vi "1830-C & CM110.vi"() -> (1 "Response":string)   [LabVIEW 2012]
doc: "This VI allows the user to communicate with the 1835-C through the GPIB bus. If the command sent is a query, the VI will automatically read the response. This VI also checks for errors and lets the user know if one exists."
panel:
  out "millisecond timer value":u32
  out "Message String 4":string
  out "1830-C Label on top. 4":string="Optical Power Meter     Model 1830-C"
  out "Power":string
  out "488 Timeout 4":i32
  in  "time delay  2":u32=6000
  out "status byte 2":u8
  out "cancel byte  2":u8 step=1
  out "timeout  2":bool
  in  "NEW GRT?":u8=1 min=1 max=2 step=1
  in  "port number  2":T1(ring)
  in  "1830-C GPIB Address 2":i16=4
  out "1830-C Label on top. 2":string="Optical Power Meter     Model 1830-C"
  out "error out":errorcluster
  in  "error in (no error)":errorcluster
  in  "File":path
  out "Message String 3":string
  out "Wavelength":string
  out "488 Timeout 3":i32
  out "String":string
  in  "WAVELENGTH":u16
  in  "time delay":u32=20000
  out "status byte":u8
  out "cancel byte":u8
  out "timeout":bool
  in  "port number":T1(ring)
  out "488 Timeout":i32
  out "Message String":string
  out "1830-C Label on top.":string="Optical Power Meter     Model 1830-C"
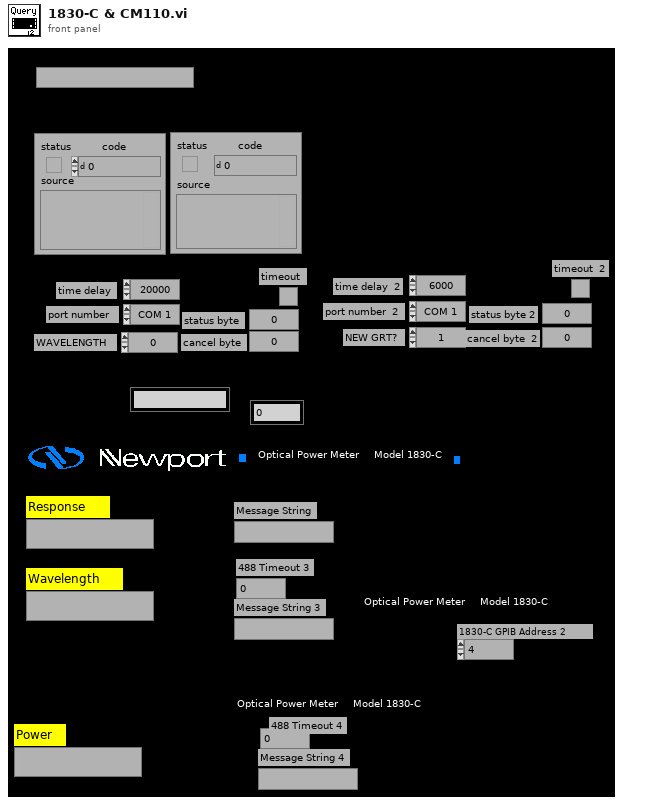
[diagram p1: front panel]
types:
  T1 = enum8{"COM 1", "COM 2", "COM 3", "COM 4", "COM 5", "COM 6", "COM 7", "COM 8", "COM 9"}
  T2 = enum16{"open", "replace", "create", "open or create", "replace or create", "replace or create with confirmation"}
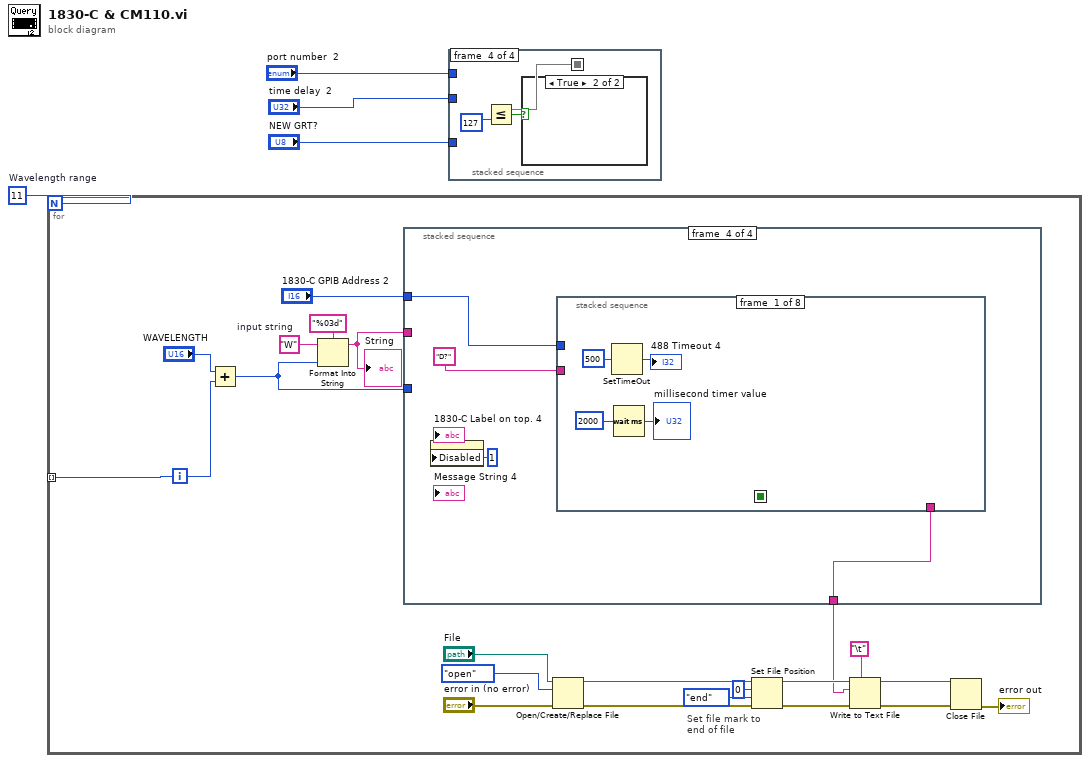
[diagram p0: block diagram]
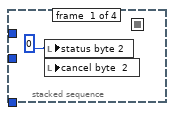
[diagram p2: hidden frame]
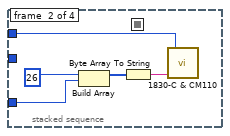
[diagram p3: hidden frame]
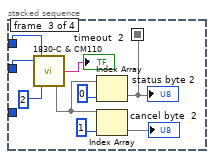
[diagram p4: hidden frame]
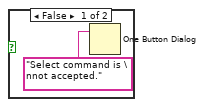
[diagram p5: hidden frame]
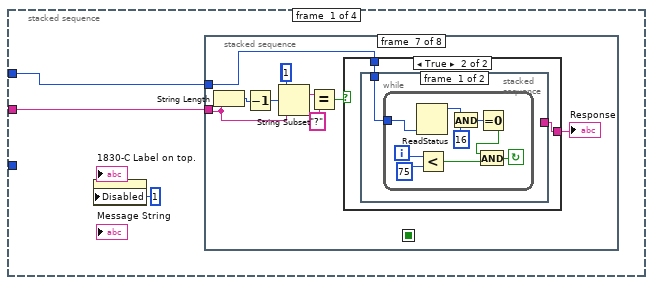
[diagram p6: hidden frame]
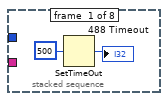
[diagram p7: hidden frame]
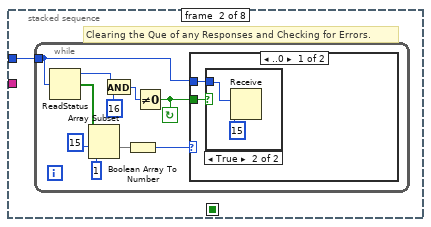
[diagram p8: hidden frame]
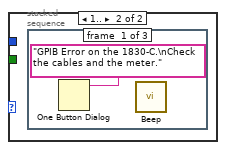
[diagram p10: hidden frame]
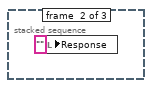
[diagram p11: hidden frame]
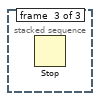
[diagram p12: hidden frame]
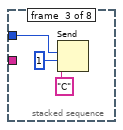
[diagram p13: hidden frame]
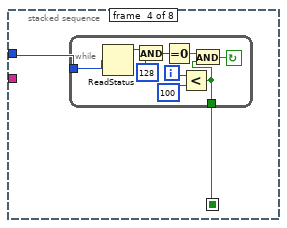
[diagram p14: hidden frame]
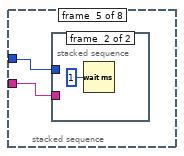
[diagram p15: hidden frame]
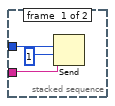
[diagram p16: hidden frame]
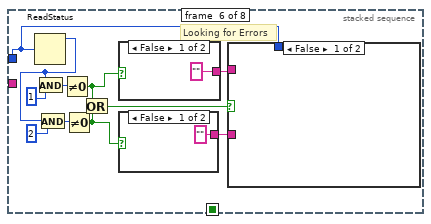
[diagram p17: hidden frame]
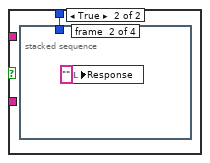
[diagram p18: hidden frame]
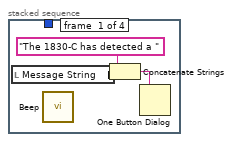
[diagram p19: hidden frame]
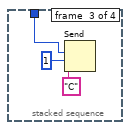
[diagram p20: hidden frame]
diagram:
  w4 = 11  # Wavelength range
  n1 = for {
    N: w4 -> [_]
    tunnel: [w21] -> _ mode=indexing
    i -> [w21]
    w25 = "W"  # input string
    # "Set file mark to\nend of file"
    n2 = Add(x="WAVELENGTH", y=w21) -> (x+y=w20:i32)
    n3 = Format Into String(format string="%03d", initial string=w25, w20) -> (resulting string=w24:string)  [unwired: 1 in, 1 out]
    "String" <- w24
    n4 = stacked-sequence {
      tunnel: w20 -> [_ w117 _ _]
      tunnel: w24 -> [w27 _ _ _]
      tunnel: [_ _ _ w233] -> w6
      tunnel: "1830-C GPIB Address 2" -> [w26 _ w141 w232]
      frame #0 {
        n5 = property on="1830-C Label on top." class="Str"("Disabled"=u8 1) -> ()  [unwired: 2 in, 2 out]
        n6 = stacked-sequence {
          seq-local: [_ _ _ w51 _ _ _ _] -> [_ _ _ _ _ _ _ _]
          tunnel: w27 -> [_ _ _ _ w62 _ w95 _]
          tunnel: w26 -> [_ w31 w49 w52 w63 w68 w99 _]
          frame #0 {
            n7 = SetTimeOut(1:500) -> (0:→"488 Timeout":i32)
          }
          frame #1 {
            # "Clearing the Que of any Responses and Checking for Errors."
            n8 = while {
              tunnel: w31 -> [w33]
              stop <- w35 continue-if-true
              n9 = ReadStatus(4:w33) -> (1:w40:bool[], 2:w34:i16)  [unwired: 2 in, 1 out]
              n10 = Array Subset(array=w40, index=15, length=1) -> (w37:bool[])
              n11 = And(x=w34, y=i16 16) -> (x .and. y?=w41:i16)
              n12 = Boolean Array To Number(Boolean array=w37) -> (number=w36:u32)
              n13 = Not Equal To 0?(x=w41) -> (x != 0?=w35:bool)
              n14 = case shown="..0" w36 {
                tunnel: w35 -> [w43 _]
                tunnel: w33 -> [w42 _]
                frame ..0 {
                  n15 = case shown="True" w43 {
                    tunnel: w42 -> [_ w45]
                    frame False {
                    }
                    frame True {
                      n16 = Receive(6:15, 8:w45) -> ()  [unwired: 3 in, 4 out]
                    }
                  }
                }
                frame 1.. {
                  n17 = stacked-sequence {
                    frame #0 {
                      n18 = One Button Dialog(message="GPIB Error on the 1830-C.\nCheck the cables and the meter.") -> ()  [unwired: 1 in, 1 out]
                      n19 = call <vilib>:"Beep.vi"() -> ()  [unwired: 12 in]
                    }
                    frame #1 {
                      n20 = local write "Response"("") -> ()
                    }
                    frame #2 {
                      n21 = Stop() -> ()  [unwired: 1 in]
                    }
                  }
                }
              }
            }
          }
          frame #2 {
            n22 = Send(2:w49, 3:u8 1, 5:"C") -> ()  [unwired: 2 in, 3 out]
          }
          frame #3 {
            n23 = while {
              tunnel: [w54] -> w51
              tunnel: w52 -> [w53]
              i -> [w57]
              stop <- w55 continue-if-true
              n24 = ReadStatus(4:w53) -> (2:w56:i16)  [unwired: 2 in, 2 out]
              n25 = And(x=w56, y=i16 128) -> (x .and. y?=w60:i16)
              n26 = Equal To 0?(x=w60) -> (x = 0?=w58:bool)
              n27 = Less?(x=w57, y=100) -> (x < y?=w54:bool)
              n28 = And(x=w58, y=w54) -> (x .and. y?=w55:bool)
            }
          }
          frame #4 {
            n29 = stacked-sequence {
              tunnel: w63 -> [w65 _]
              tunnel: w62 -> [w64 _]
              frame #0 {
                n30 = Send(2:w65, 3:u8 1, 5:w64) -> ()  [unwired: 2 in, 3 out]
              }
              frame #1 {
                n31 = Wait (ms)(milliseconds to wait=u32 1) -> ()  [unwired: 1 out]
              }
            }
          }
          frame #5 {
            # "Looking for Errors"
            n32 = ReadStatus(4:w68) -> (2:w76:i16)  [unwired: 2 in, 2 out]
            n33 = And(x=w76, y=i16 1) -> (x .and. y?=w75:i16)
            n34 = And(x=w76, y=i16 2) -> (x .and. y?=w74:i16)
            n35 = Not Equal To 0?(x=w75) -> (x != 0?=w73:bool)
            n36 = Not Equal To 0?(x=w74) -> (x != 0?=w72:bool)
            n37 = Or(x=w73, y=w72) -> (x .or. y?=w71:bool)
            n38 = case shown="False" w73 {
              tunnel: ["" w90] -> w69
              frame False {
              }
              frame True {
                w90 = "Parameter Error."
                n39 = local write "Message String"(w90) -> ()
              }
            }
            n40 = case shown="False" w72 {
              tunnel: ["" w88] -> w70
              frame False {
              }
              frame True {
                w88 = "Command Error."
                n41 = local write "Message String"(w88) -> ()
              }
            }
            n42 = case shown="False" w71 {
              tunnel: w70 -> [_ _]
              tunnel: w69 -> [_ _]
              tunnel: w68 -> [_ w79]
              frame False {
              }
              frame True {
                n43 = stacked-sequence {
                  tunnel: w79 -> [_ _ w84 _]
                  frame #0 {
                    n44 = local read "Message String"() -> (w80:string)
                    n45 = call <vilib>:"Beep.vi"() -> ()  [unwired: 12 in]
                    n46 = Concatenate Strings("The 1830-C has detected a ", w80) -> (w82:string)
                    n47 = One Button Dialog(message=w82) -> ()  [unwired: 1 in, 1 out]
                  }
                  frame #1 {
                    n48 = local write "Response"("") -> ()
                  }
                  frame #2 {
                    n49 = Send(2:w84, 3:u8 1, 5:"C") -> ()  [unwired: 2 in, 3 out]
                  }
                  frame #3 {
                    n50 = Stop() -> ()  [unwired: 1 in]
                  }
                }
              }
            }
          }
          frame #6 {
            (unwired) 1
            n51 = String Length(string=w95) -> (length=w97:i32)
            n52 = Decrement(x=w97) -> (x-1=w96:i32)
            n53 = String Subset(string=w95, offset (0)=w96, length (rest)=1) -> (substring=w94:string)
            n54 = Equal?(x=w94, y="?") -> (x = y?=w92:bool)
            n55 = case shown="True" w92 {
              tunnel: w99 -> [_ w102]
              tunnel: ["" w101] -> w98
              frame False {
              }
              frame True {
                n56 = stacked-sequence {
                  tunnel: w102 -> [w103 w114]
                  tunnel: [_ w113] -> w101
                  frame #0 {
                    n57 = while {
                      tunnel: w103 -> [w109]
                      i -> [w108]
                      stop <- w104 continue-if-true
                      n58 = ReadStatus(4:w109) -> (2:w110:i16)  [unwired: 2 in, 2 out]
                      n59 = Less?(x=w108, y=75) -> (x < y?=w105:bool)
                      n60 = And(x=w110, y=i16 16) -> (x .and. y?=w111:i16)
                      n61 = Equal To 0?(x=w111) -> (x = 0?=w106:bool)
                      n62 = And(x=w106, y=w105) -> (x .and. y?=w104:bool)
                    }
                  }
                  frame #1 {
                    n63 = Receive(6:15, 8:w114) -> (3:w113:string)  [unwired: 3 in, 3 out]
                  }
                }
              }
            }
            "Response" <- w98
          }
          frame #7 {
            n64 = local read "488 Timeout"() -> (w116:i32)
            n65 = SetTimeOut(1:w116) -> ()  [unwired: 1 out]
          }
        }
      }
      frame #1 {
        n66 = stacked-sequence {
          seq-local: [_ _ w131 _] -> [_ _ _ w139]
          tunnel: w117 -> [_ w127 _ _]
          tunnel: "port number" -> [_ w121 w128 _]
          tunnel: "time delay" -> [_ _ w130 _]
          frame #0 {
            w120 = u8 0
            n67 = local write "status byte"(w120) -> ()
            n68 = local write "cancel byte"(w120) -> ()
          }
          frame #1 {
            n69 = Split Number(x=w127) -> (hi(x)=w126:u16, lo(x)=w125:u16)
            n70 = Build Array(u8 16, w126, w125) -> (w123:u16[])
            n71 = Byte Array To String(unsigned byte array=w123) -> (string=w122:string)
            n72 = call "1830-C & CM110.vi"("string to write"=w122, "port number"=w121) -> ()  [unwired: 1 out]
          }
          frame #2 {
            n73 = call "1830-C & CM110.vi"(3:2, 4:w130, 5:w128) -> (0:w133, "Response"=→"timeout":string)  [unwired: 1 in]
            n74 = Index Array(array=w133, index=0) -> (element=w131)
            "status byte" <- w131
            n75 = Index Array(array=w133, index=1) -> (element=→"cancel byte")
          }
          frame #3 {
            n76 = Less Or Equal?(x=w139, y=127) -> (x <= y?=w137:bool)
            n77 = case shown="True" w137 {
              frame False {
                n78 = One Button Dialog(message="Goto command is \nnot accepted.") -> ()  [unwired: 1 in, 1 out]
              }
              frame True {
              }
            }
          }
        }
      }
      frame #2 {
        n79 = property on="1830-C Label on top. 2" class="Str"("Disabled"=u8 1) -> ()  [unwired: 2 in, 2 out]
        n80 = stacked-sequence {
          seq-local: [_ _ _ w166 _ _ _ _] -> [_ _ _ _ _ _ _ _]
          tunnel: "W?" ("Single Command/Query 3") -> [_ _ _ _ w177 _ w211 _]
          tunnel: w141 -> [_ w146 w164 w167 w178 w183 w214 _]
          frame #0 {
            n81 = SetTimeOut(1:500) -> (0:→"488 Timeout 3":i32)
          }
          frame #1 {
            # "Clearing the Que of any Responses and Checking for Errors."
            n82 = while {
              tunnel: w146 -> [w148]
              stop <- w150 continue-if-true
              n83 = ReadStatus(4:w148) -> (1:w155:bool[], 2:w149:i16)  [unwired: 2 in, 1 out]
              n84 = Array Subset(array=w155, index=15, length=1) -> (w152:bool[])
              n85 = And(x=w149, y=i16 16) -> (x .and. y?=w156:i16)
              n86 = Boolean Array To Number(Boolean array=w152) -> (number=w151:u32)
              n87 = Not Equal To 0?(x=w156) -> (x != 0?=w150:bool)
              n88 = case shown="..0" w151 {
                tunnel: w150 -> [w158 _]
                tunnel: w148 -> [w157 _]
                frame ..0 {
                  n89 = case shown="False" w158 {
                    tunnel: w157 -> [_ w160]
                    frame False {
                    }
                    frame True {
                      n90 = Receive(6:15, 8:w160) -> ()  [unwired: 3 in, 4 out]
                    }
                  }
                }
                frame 1.. {
                  n91 = stacked-sequence {
                    frame #0 {
                      n92 = One Button Dialog(message="GPIB Error on the 1830-C.\nCheck the cables and the meter.") -> ()  [unwired: 1 in, 1 out]
                      n93 = call <vilib>:"Beep.vi"() -> ()  [unwired: 12 in]
                    }
                    frame #1 {
                      n94 = local write "Wavelength"("") -> ()
                    }
                    frame #2 {
                      n95 = Stop() -> ()  [unwired: 1 in]
                    }
                  }
                }
              }
            }
          }
          frame #2 {
            n96 = Send(2:w164, 3:u8 1, 5:"C") -> ()  [unwired: 2 in, 3 out]
          }
          frame #3 {
            n97 = while {
              tunnel: [w169] -> w166
              tunnel: w167 -> [w168]
              i -> [w172]
              stop <- w170 continue-if-true
              n98 = ReadStatus(4:w168) -> (2:w171:i16)  [unwired: 2 in, 2 out]
              n99 = And(x=w171, y=i16 128) -> (x .and. y?=w175:i16)
              n100 = Equal To 0?(x=w175) -> (x = 0?=w173:bool)
              n101 = Less?(x=w172, y=100) -> (x < y?=w169:bool)
              n102 = And(x=w173, y=w169) -> (x .and. y?=w170:bool)
            }
          }
          frame #4 {
            n103 = stacked-sequence {
              tunnel: w178 -> [w180 _]
              tunnel: w177 -> [w179 _]
              frame #0 {
                n104 = Send(2:w180, 3:u8 1, 5:w179) -> ()  [unwired: 2 in, 3 out]
              }
              frame #1 {
                n105 = Wait (ms)(milliseconds to wait=u32 1) -> ()  [unwired: 1 out]
              }
            }
          }
          frame #5 {
            # "Looking for Errors"
            n106 = ReadStatus(4:w183) -> (2:w191:i16)  [unwired: 2 in, 2 out]
            n107 = And(x=w191, y=i16 1) -> (x .and. y?=w190:i16)
            n108 = And(x=w191, y=i16 2) -> (x .and. y?=w189:i16)
            n109 = Not Equal To 0?(x=w190) -> (x != 0?=w188:bool)
            n110 = Not Equal To 0?(x=w189) -> (x != 0?=w187:bool)
            n111 = Or(x=w188, y=w187) -> (x .or. y?=w186:bool)
            n112 = case shown="False" w188 {
              tunnel: ["" w205] -> w184
              frame False {
              }
              frame True {
                w205 = "Parameter Error."
                n113 = local write "Message String 3"(w205) -> ()
              }
            }
            n114 = case shown="False" w187 {
              tunnel: ["" w203] -> w185
              frame False {
              }
              frame True {
                w203 = "Command Error."
                n115 = local write "Message String 3"(w203) -> ()
              }
            }
            n116 = case shown="False" w186 {
              tunnel: w185 -> [_ _]
              tunnel: w184 -> [_ _]
              tunnel: w183 -> [_ w194]
              frame False {
              }
              frame True {
                n117 = stacked-sequence {
                  tunnel: w194 -> [_ _ w199 _]
                  frame #0 {
                    n118 = local read "Message String 3"() -> (w195:string)
                    n119 = call <vilib>:"Beep.vi"() -> ()  [unwired: 12 in]
                    n120 = Concatenate Strings("The 1830-C has detected a ", w195) -> (w197:string)
                    n121 = One Button Dialog(message=w197) -> ()  [unwired: 1 in, 1 out]
                  }
                  frame #1 {
                    n122 = local write "Wavelength"("") -> ()
                  }
                  frame #2 {
                    n123 = Send(2:w199, 3:u8 1, 5:"C") -> ()  [unwired: 2 in, 3 out]
                  }
                  frame #3 {
                    n124 = Stop() -> ()  [unwired: 1 in]
                  }
                }
              }
            }
          }
          frame #6 {
            (unwired) 1
            n125 = String Length(string=w211) -> (length=w213:i32)
            n126 = Decrement(x=w213) -> (x-1=w212:i32)
            n127 = String Subset(string=w211, offset (0)=w212, length (rest)=1) -> (substring=w210:string)
            n128 = Equal?(x=w210, y="?") -> (x = y?=w208:bool)
            n129 = case shown="True" w208 {
              tunnel: w214 -> [_ w217]
              tunnel: ["" w216] -> w206
              frame False {
              }
              frame True {
                n130 = stacked-sequence {
                  tunnel: w217 -> [w218 w229]
                  tunnel: [_ w228] -> w216
                  frame #0 {
                    n131 = while {
                      tunnel: w218 -> [w224]
                      i -> [w223]
                      stop <- w219 continue-if-true
                      n132 = ReadStatus(4:w224) -> (2:w225:i16)  [unwired: 2 in, 2 out]
                      n133 = Less?(x=w223, y=75) -> (x < y?=w220:bool)
                      n134 = And(x=w225, y=i16 16) -> (x .and. y?=w226:i16)
                      n135 = Equal To 0?(x=w226) -> (x = 0?=w221:bool)
                      n136 = And(x=w221, y=w220) -> (x .and. y?=w219:bool)
                    }
                  }
                  frame #1 {
                    n137 = Receive(6:15, 8:w229) -> (3:w228:string)  [unwired: 3 in, 3 out]
                  }
                }
              }
            }
            "Wavelength" <- w206
          }
          frame #7 {
            n138 = local read "488 Timeout 3"() -> (w231:i32)
            n139 = SetTimeOut(1:w231) -> ()  [unwired: 1 out]
          }
        }
      }
      frame #3 {
        n140 = property on="1830-C Label on top. 4" class="Str"("Disabled"=u8 1) -> ()  [unwired: 2 in, 2 out]
        n141 = stacked-sequence {
          seq-local: [_ _ _ w260 _ _ _ _] -> [_ _ _ _ _ _ _ _]
          tunnel: "D?" ("Single Command/Query 2") -> [_ _ _ _ w271 _ w305 _]
          tunnel: w232 -> [_ w240 w258 w261 w272 w277 w308 _]
          tunnel: [_ _ _ _ _ _ w300 _] -> w233
          frame #0 {
            n142 = SetTimeOut(1:500) -> (0:→"488 Timeout 4":i32)
            n143 = Wait (ms)(milliseconds to wait=2000) -> (millisecond timer value=→"millisecond timer value":u32)
          }
          frame #1 {
            # "Clearing the Que of any Responses and Checking for Errors."
            n144 = while {
              tunnel: w240 -> [w242]
              stop <- w244 continue-if-true
              n145 = ReadStatus(4:w242) -> (1:w249:bool[], 2:w243:i16)  [unwired: 2 in, 1 out]
              n146 = Array Subset(array=w249, index=15, length=1) -> (w246:bool[])
              n147 = And(x=w243, y=i16 16) -> (x .and. y?=w250:i16)
              n148 = Boolean Array To Number(Boolean array=w246) -> (number=w245:u32)
              n149 = Not Equal To 0?(x=w250) -> (x != 0?=w244:bool)
              n150 = case shown="..0" w245 {
                tunnel: w244 -> [w252 _]
                tunnel: w242 -> [w251 _]
                frame ..0 {
                  n151 = case shown="False" w252 {
                    tunnel: w251 -> [_ w254]
                    frame False {
                    }
                    frame True {
                      n152 = Receive(6:15, 8:w254) -> ()  [unwired: 3 in, 4 out]
                    }
                  }
                }
                frame 1.. {
                  n153 = stacked-sequence {
                    frame #0 {
                      n154 = One Button Dialog(message="GPIB Error on the 1830-C.\nCheck the cables and the meter.") -> ()  [unwired: 1 in, 1 out]
                      n155 = call <vilib>:"Beep.vi"() -> ()  [unwired: 12 in]
                    }
                    frame #1 {
                      n156 = local write "Power"("") -> ()
                    }
                    frame #2 {
                      n157 = Stop() -> ()  [unwired: 1 in]
                    }
                  }
                }
              }
            }
          }
          frame #2 {
            n158 = Send(2:w258, 3:u8 1, 5:"C") -> ()  [unwired: 2 in, 3 out]
          }
          frame #3 {
            n159 = while {
              tunnel: [w263] -> w260
              tunnel: w261 -> [w262]
              i -> [w266]
              stop <- w264 continue-if-true
              n160 = ReadStatus(4:w262) -> (2:w265:i16)  [unwired: 2 in, 2 out]
              n161 = And(x=w265, y=i16 128) -> (x .and. y?=w269:i16)
              n162 = Equal To 0?(x=w269) -> (x = 0?=w267:bool)
              n163 = Less?(x=w266, y=100) -> (x < y?=w263:bool)
              n164 = And(x=w267, y=w263) -> (x .and. y?=w264:bool)
            }
          }
          frame #4 {
            n165 = stacked-sequence {
              tunnel: w272 -> [w274 _]
              tunnel: w271 -> [w273 _]
              frame #0 {
                n166 = Send(2:w274, 3:u8 1, 5:w273) -> ()  [unwired: 2 in, 3 out]
              }
              frame #1 {
                n167 = Wait (ms)(milliseconds to wait=u32 1) -> ()  [unwired: 1 out]
              }
            }
          }
          frame #5 {
            # "Looking for Errors"
            n168 = ReadStatus(4:w277) -> (2:w285:i16)  [unwired: 2 in, 2 out]
            n169 = And(x=w285, y=i16 1) -> (x .and. y?=w284:i16)
            n170 = And(x=w285, y=i16 2) -> (x .and. y?=w283:i16)
            n171 = Not Equal To 0?(x=w284) -> (x != 0?=w282:bool)
            n172 = Not Equal To 0?(x=w283) -> (x != 0?=w281:bool)
            n173 = Or(x=w282, y=w281) -> (x .or. y?=w280:bool)
            n174 = case shown="False" w282 {
              tunnel: ["" w299] -> w278
              frame False {
              }
              frame True {
                w299 = "Parameter Error."
                n175 = local write "Message String 4"(w299) -> ()
              }
            }
            n176 = case shown="False" w281 {
              tunnel: ["" w297] -> w279
              frame False {
              }
              frame True {
                w297 = "Command Error."
                n177 = local write "Message String 4"(w297) -> ()
              }
            }
            n178 = case shown="False" w280 {
              tunnel: w279 -> [_ _]
              tunnel: w278 -> [_ _]
              tunnel: w277 -> [_ w288]
              frame False {
              }
              frame True {
                n179 = stacked-sequence {
                  tunnel: w288 -> [_ _ w293 _]
                  frame #0 {
                    n180 = local read "Message String 4"() -> (w289:string)
                    n181 = call <vilib>:"Beep.vi"() -> ()  [unwired: 12 in]
                    n182 = Concatenate Strings("The 1830-C has detected a ", w289) -> (w291:string)
                    n183 = One Button Dialog(message=w291) -> ()  [unwired: 1 in, 1 out]
                  }
                  frame #1 {
                    n184 = local write "Power"("") -> ()
                  }
                  frame #2 {
                    n185 = Send(2:w293, 3:u8 1, 5:"C") -> ()  [unwired: 2 in, 3 out]
                  }
                  frame #3 {
                    n186 = Stop() -> ()  [unwired: 1 in]
                  }
                }
              }
            }
          }
          frame #6 {
            n187 = String Length(string=w305) -> (length=w307:i32)
            n188 = Decrement(x=w307) -> (x-1=w306:i32)
            n189 = String Subset(string=w305, offset (0)=w306, length (rest)=1) -> (substring=w304:string)
            n190 = Equal?(x=w304, y="?") -> (x = y?=w302:bool)
            n191 = case shown="True" w302 {
              tunnel: w308 -> [_ w311]
              tunnel: ["" w310] -> w300
              frame False {
              }
              frame True {
                n192 = stacked-sequence {
                  tunnel: w311 -> [w312 w323]
                  tunnel: [_ w322] -> w310
                  frame #0 {
                    n193 = while {
                      tunnel: w312 -> [w318]
                      i -> [w317]
                      stop <- w313 continue-if-true
                      n194 = ReadStatus(4:w318) -> (2:w319:i16)  [unwired: 2 in, 2 out]
                      n195 = Less?(x=w317, y=75) -> (x < y?=w314:bool)
                      n196 = And(x=w319, y=i16 16) -> (x .and. y?=w320:i16)
                      n197 = Equal To 0?(x=w320) -> (x = 0?=w315:bool)
                      n198 = And(x=w315, y=w314) -> (x .and. y?=w313:bool)
                    }
                  }
                  frame #1 {
                    n199 = Receive(6:15, 8:w323) -> (3:w322:string)  [unwired: 3 in, 3 out]
                  }
                }
              }
            }
            "Power" <- w300
          }
          frame #7 {
            n200 = local read "488 Timeout 4"() -> (w325:i32)
            n201 = SetTimeOut(1:w325) -> ()  [unwired: 1 out]
          }
        }
      }
    }
    n202 = Open/Create/Replace File(file path (use dialog)="File", error in="error in (no error)", operation (0:open)=T2."open") -> (refnum out=w11:refnum<file>, error out=w10:errorcluster)  [unwired: 3 in, 1 out]
    n203 = Set File Position(offset (in bytes) (0)=i64 0, refnum=w11, from (0:start)=enum16{"start", "end", "current"}."end", error in=w10) -> (refnum out=w15:refnum<file>, error out=w16:errorcluster)
    n204 = Write to Text File(prompt (Choose or enter file path)="\t", file (use dialog)=w15, text=w6, error in=w16) -> (refnum out=w13:refnum<file>, error out=w14:errorcluster)  [unwired: 1 out]
    n205 = Close File(refnum=w13, error in=w14) -> (error out=→"error out":errorcluster)  [unwired: 1 out]
  }
  n206 = stacked-sequence {
    seq-local: [_ _ w335 _] -> [_ _ _ w343]
    tunnel: "port number  2" -> [_ w327 w332 _]
    tunnel: "time delay  2" -> [_ _ w334 _]
    tunnel: "NEW GRT?" -> [_ w328 _ _]
    frame #0 {
      w326 = u8 0
      n207 = local write "status byte 2"(w326) -> ()
      n208 = local write "cancel byte  2"(w326) -> ()
    }
    frame #1 {
      n209 = Build Array(u8 26, w328) -> (w330:u8[])
      n210 = Byte Array To String(unsigned byte array=w330) -> (string=w329:string)
      n211 = call "1830-C & CM110.vi"("string to write"=w329, "port number"=w327) -> ()  [unwired: 1 out]
    }
    frame #2 {
      n212 = call "1830-C & CM110.vi"(3:2, 4:w334, 5:w332) -> (0:w337, "Response"=→"timeout  2":string)  [unwired: 1 in]
      n213 = Index Array(array=w337, index=0) -> (element=w335)
      "status byte 2" <- w335
      n214 = Index Array(array=w337, index=1) -> (element=→"cancel byte  2")
    }
    frame #3 {
      n215 = Less Or Equal?(x=w343, y=127) -> (x <= y?=w341:bool)
      n216 = case shown="True" w341 {
        frame False {
          n217 = One Button Dialog(message="Select command is \nnot accepted.") -> ()  [unwired: 1 in, 1 out]
        }
        frame True {
        }
      }
    }
  }
